vi "ANAL_DeriveDataHelper.vi"(0 "Run Info Out":T2, 5 "Run Data Cluster":T1 {"Temperature B" scale=0.0..100.0; "Temperature A" scale=0.0..100.0}) -> (4 "Run Info Out 2":T2, 6 "Run Data Cluster 2":T1 {"Temperature B" scale=0.0..100.0; "Temperature A" scale=0.0..100.0}, 8 "No. Sweeps":i32, 10 "Delta":dbl, 13 "Temp Range":string, 14 "Ampl Range":string, 15 "End Time":timestamp)   [LabVIEW 2021]
uses:
  XML_Cluster.ctl
  DAT_Cluster.ctl
  ff163555-c4eb-45d0-9485-ef42e3709eca.vi
  <vilib>/Analysis/baseanly.llb/Mean (DBL).vi
  <vilib>/Comparison/Less/Less Functor/Less Functor.lvclass
  <vilib>/Analysis/NI_AALBase.lvlib
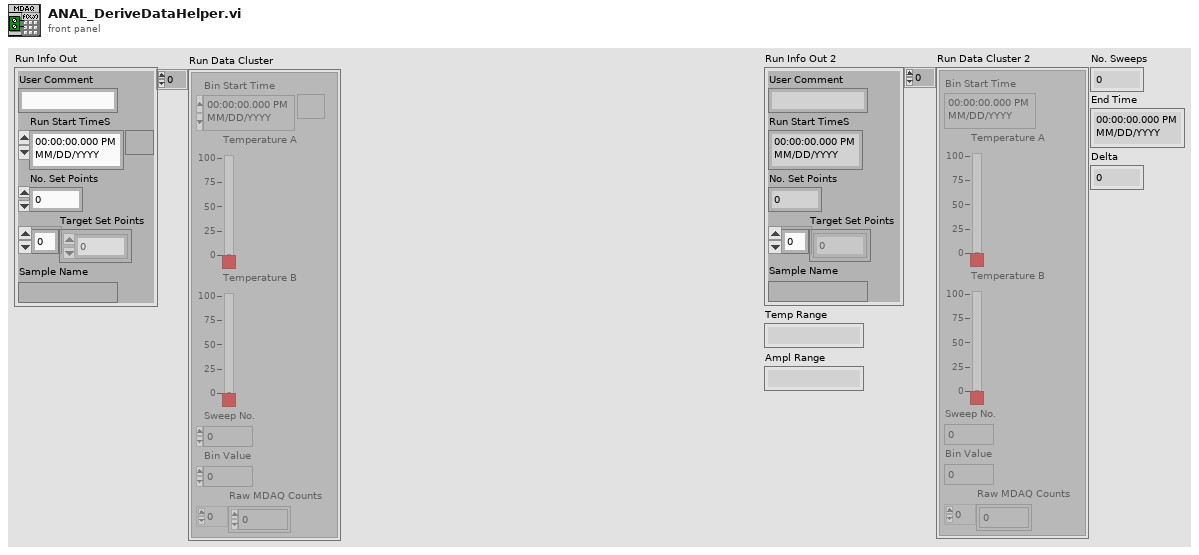
[diagram p1: front panel]
types:
  T1 = typedef "DAT_Cluster.ctl" = cluster{"Bin Start Time":timestamp, "Temperature A":dbl, "Temperature B":dbl, "Sweep No.":i32, "Bin Value":i32, "Raw MDAQ Counts":i32[]}[]
  T2 = typedef "XML_Cluster.ctl" = cluster{"User Comment":string, "Run Start TimeS":timestamp, "No. Set Points":u32, "Target Set Points":i32[], "Sample Name":string}
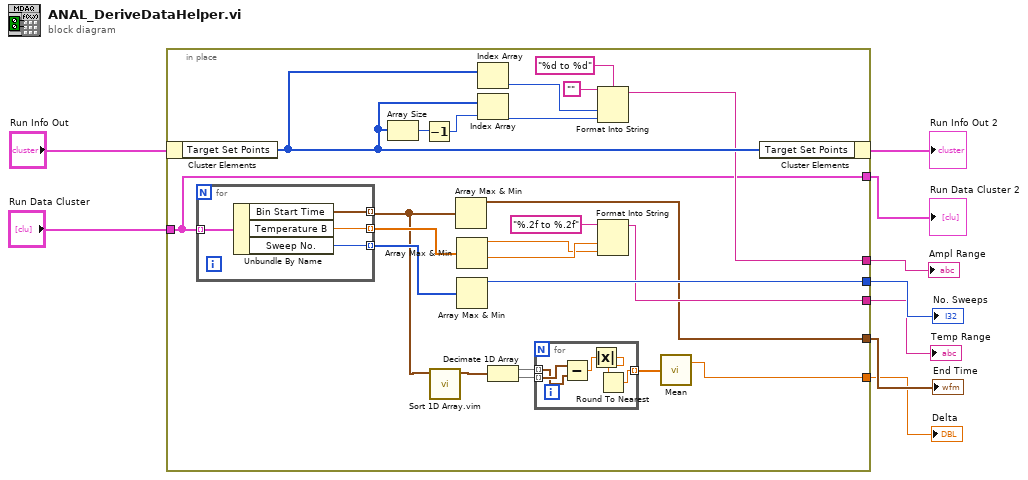
[diagram p0: block diagram]
diagram:
  n1 = in-place {
    in-place-border: "Run Data Cluster" -> [w22]
    in-place-border: [w25] -> w1
    in-place-border: [w22] -> w6
    in-place-border: [w21] -> w5
    in-place-border: [w17] -> w4
    in-place-border: [w16] -> w3
    in-place-border: [w12] -> w2
    n2 = in-place-cluster #1("Run Info Out") -> ("Target Set Points"=w30:i32[])
    n3 = for {
      tunnel: w22 -> [w41] mode=indexing
      tunnel: [w40] -> w11 mode=indexing
      tunnel: [w39] -> w24 mode=indexing
      tunnel: [w38] -> w23 mode=indexing
      n4 = Unbundle By Name(w41) -> ("Bin Start Time"=w40:timestamp, "Temperature B"=w39:dbl, "Sweep No."=w38:i32)
    }
    n5 = Array Size(array=w30) -> (size(s)=w32:i32)
    n6 = Decrement(x=w32) -> (x-1=w31:i32)
    n7 = call "Sort 1D Array.vim"("unsorted array"=w11) -> ("sorted array"=w10:timestamp[])  [unwired: 10 in]
    n8 = Array Max & Min(array=w11) -> (max value=w16:timestamp)  [unwired: 3 out]
    n9 = Array Max & Min(array=w24) -> (max value=w18:dbl, min value=w19:dbl)  [unwired: 2 out]
    n10 = Array Max & Min(array=w23) -> (max value=w21:i32)  [unwired: 3 out]
    n11 = Index Array(array=w30) -> (element=w27:i32)  [unwired: 1 in]
    n12 = Index Array(array=w30, index=w31) -> (element=w26:i32)
    n13 = Decimate 1D Array(w10) -> (w15:timestamp[], w14:timestamp[])
    n14 = for {
      tunnel: w15 -> [w36] mode=indexing
      tunnel: w14 -> [w37] mode=indexing
      tunnel: [w33] -> w13 mode=indexing
      n15 = Subtract(x=w37, y=w36) -> (x-y=w35:dbl)
      n16 = Absolute Value(x=w35) -> (abs(x)=w34:dbl)
      n17 = Round To Nearest(number=w34) -> (nearest integer value=w33:dbl)
    }
    n18 = Format Into String(format string="%d to %d", initial string="", w27, w26) -> (resulting string=w25:string)  [unwired: 1 in, 1 out]
    n19 = Format Into String(format string="%.2f to %.2f", w19, w18) -> (resulting string=w17:string)  [unwired: 2 in, 1 out]
    n20 = call-poly <vilib>:"Mean.vi"("X"=w13) -> ("mean"=w12:dbl)  [unwired: 1 out]
    n21 = in-place-cluster #1("Target Set Points"=w30) -> (→"Run Info Out 2":T2)
  }
  "Run Data Cluster 2" <- w6
  "No. Sweeps" <- w5
  "Temp Range" <- w4
  "End Time" <- w3
  "Delta" <- w2
  "Ampl Range" <- w1
